vi "FPGA Host.vi"() -> (8 "FilePath":path=path "D:/temp/test.tdms")   [LabVIEW 2023]
uses:
  TypeDefs/WayPointCluster.ctl
  TypeDefs/Settings.ctl
  TypeDefs/ChangeOnFly.ctl
  TypeDefs/Display.ctl
  <vilib>/userDefined/High Color/nirio_resource_hc.ctl
  User_Vi/Settings.vi
  <vilib>/FPGAPlugInAG/PCIe-7856/niLvFpga_Open_PCIe-7856.vi
  <vilib>/FPGAPlugInAG/PCIe-7856/niLvFpga_Run_PCIe-7856.vi
  <vilib>/Utility/error.llb/Error Cluster From Error Code.vi
  <vilib>/rvi/errors/niLvFpgaAdjustHostInterfaceError.vi
  I32NonDim_to_umNonDim.vi
  <vilib>/rvi/interface/nirviOpenFPGA/nirviOpenFPGA.xnode
  TypeDefs/FPGA VI reference.ctl
  FPGA Bitfiles/wecspmpcie7856mi_FPGATarget2_FPGATargetPCIe78_PFpA9M1zUPQ.lvbitx
  <vilib>/rvi/interface/nirviMethod/nirviMethod.xnode
  <vilib>/rvi/interface/nirviReadWriteControl/nirviReadWriteControl.xnode
  <vilib>/rvi/errors/niLvFpgaMergeErrorWithErrorCode.vi
  NiFpgaLv.dll
  <vilib>/FPGAPlugInAG/PCIe-7856/niLvFpga_WriteFifo_PCIe-7856.vi
  <vilib>/FPGAPlugInAG/PCIe-7856/niLvFpga_ReadFifo_PCIe-7856.vi
  <vilib>/FPGAPlugInAG/PCIe-7856/niLvFpga_StartFifo_PCIe-7856.vi
  <vilib>/FPGAPlugInAG/PCIe-7856/niLvFpga_StopFifo_PCIe-7856.vi
panel:
  out "output cluster":T1
  out "DistanceToBulk":i16
  out "StopMoveV2":bool
  out "StopMoveV":bool
  out "StopMoveZ":bool
  out "StopMoveY":bool
  out "StopMoveX":bool
  out "Stop Hold Position":bool
  out "HoldTimer (ticks)":u64
  out "Feedback1 on  Hold":bool
  out "MeasuredCurrent":i16
  out "LineNumber":u64
  out "Feedback_Threshold":i32
  out "Feedback1 Error":i32
  out "Feedback1 Boolean":bool
  in  "Display Cluster":T2
  in  "ChangeonFly":T3
  in  "SettingsCluster":T4={"Sample Rate (us)"=1, "Samples Per Data Point (int, power of 2)"=1000, "DistanceToBulk (um)"=-1.0, "HoldTimeScaler"=1, "SaveData"=TRUE, "DistanceToBulk (um) 2"=-1.0, "DistanceToBulk (um) 3"=-1.0}
  in  "WayPointCluster":T5
  out "tdms file out":refnum<k34>
  out "ElementsToRead":u32=800
  in  "stop":bool
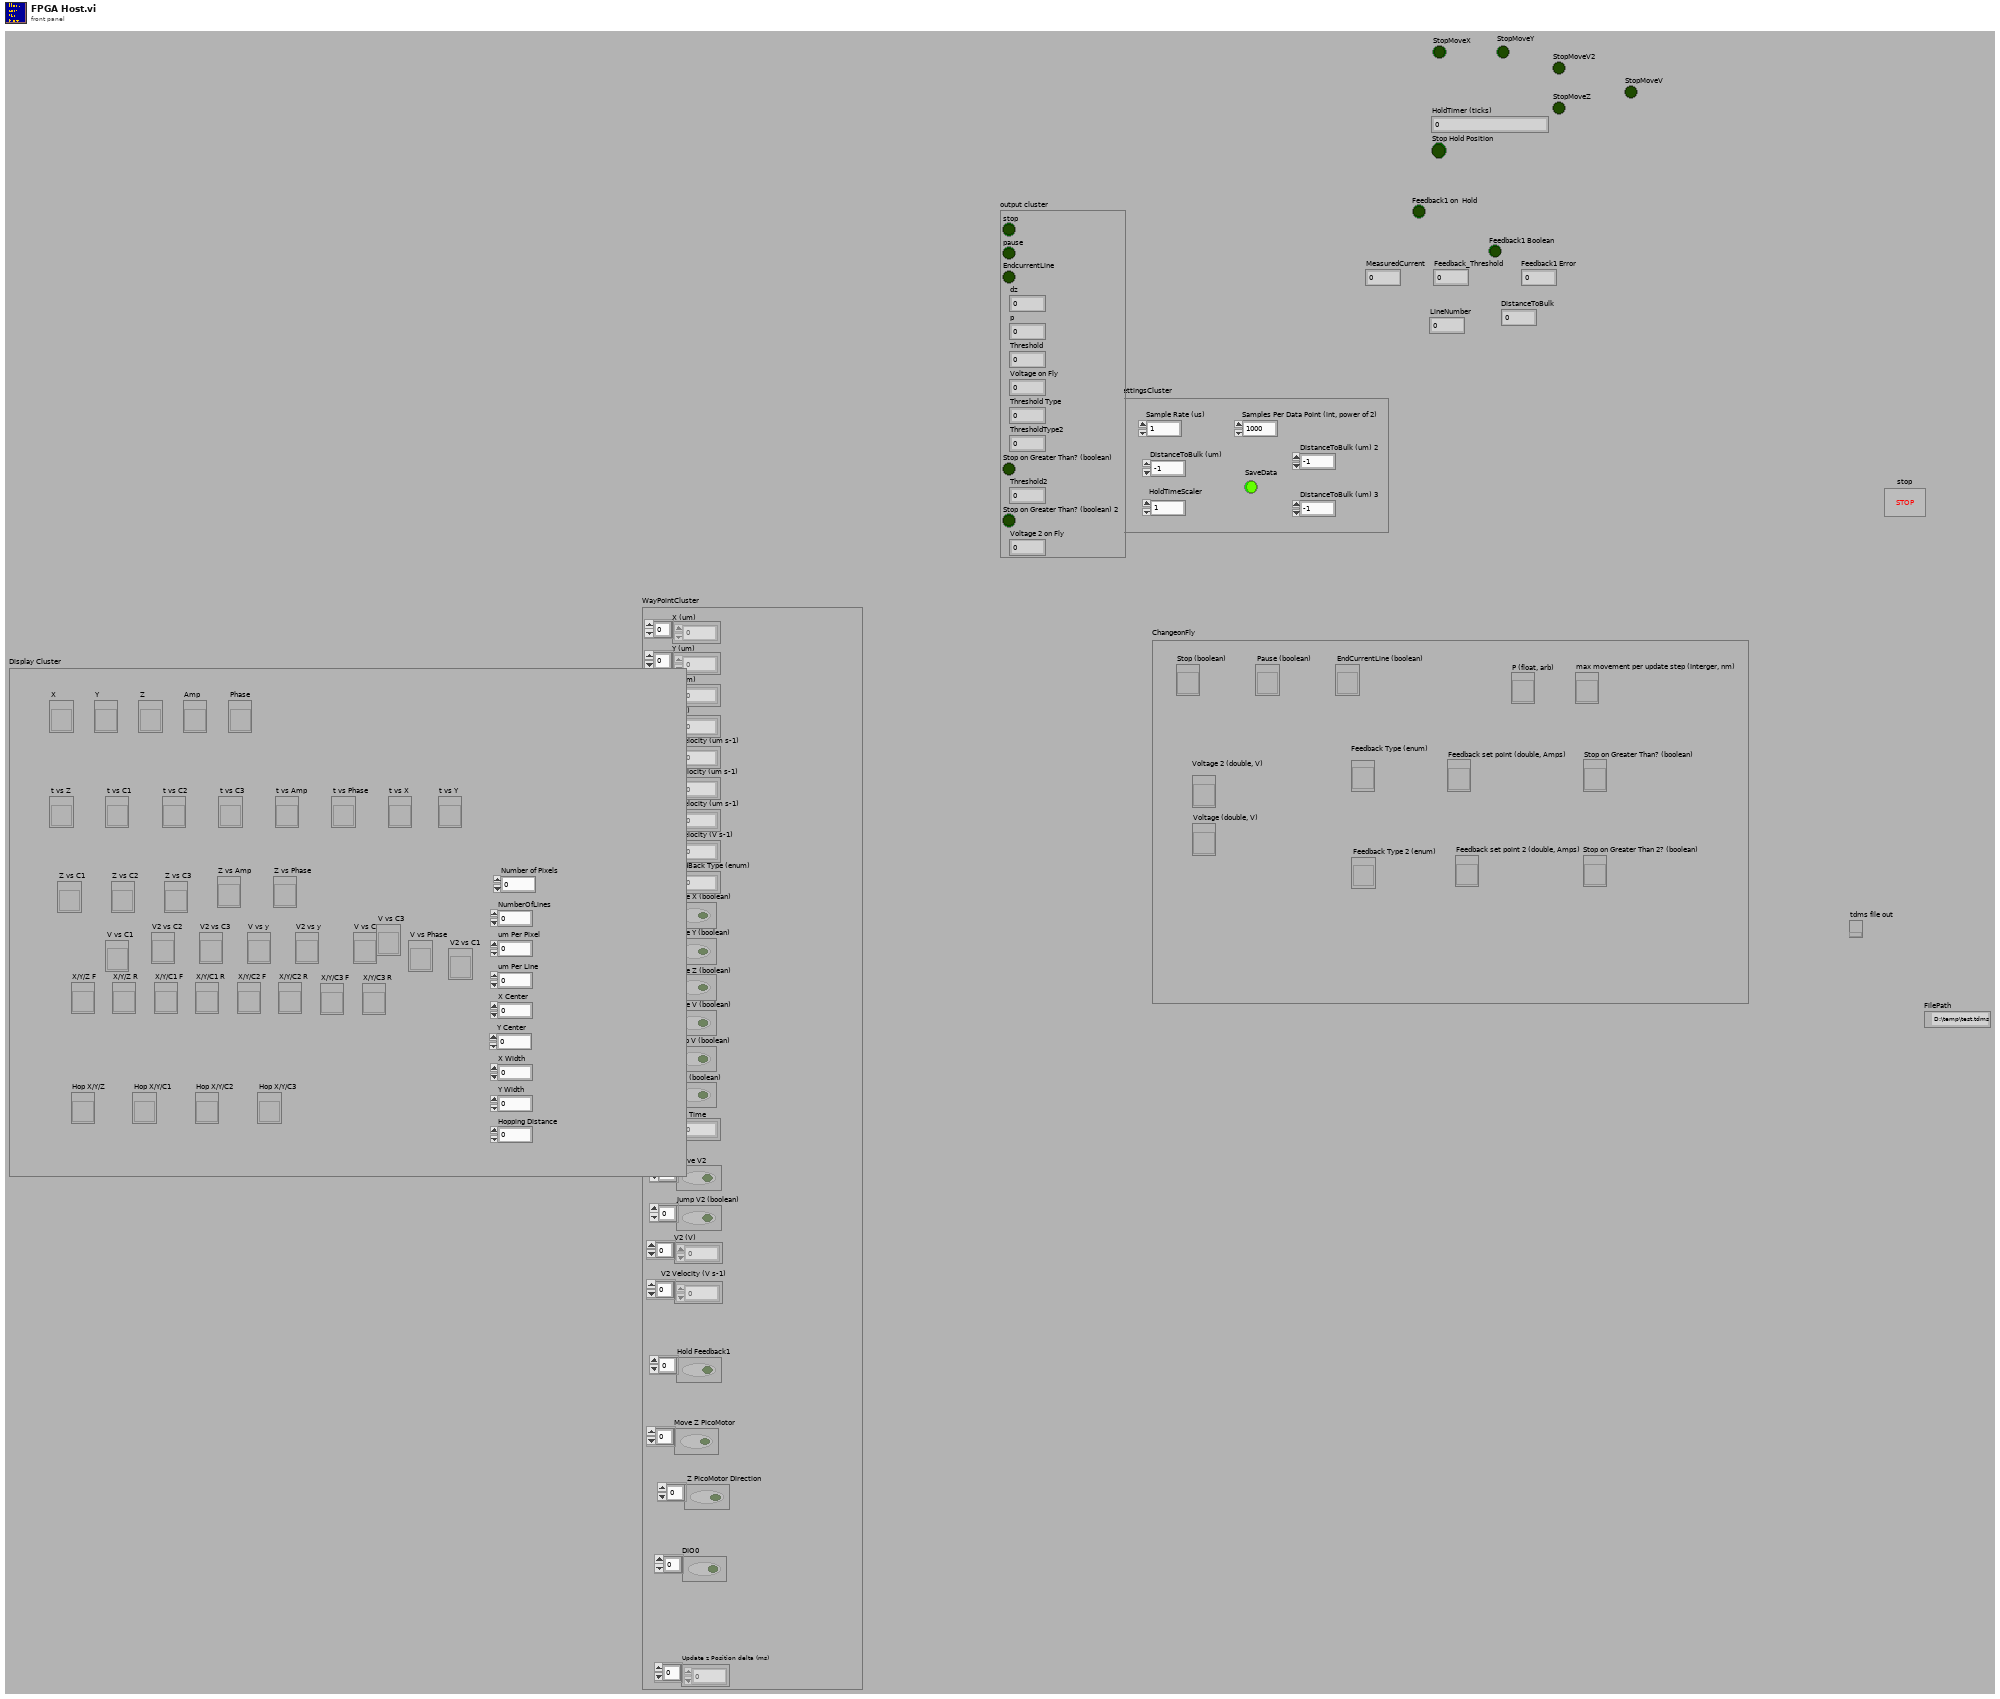
[diagram p1: front panel]
types:
  T1 = cluster{"stop":bool, "pause":bool, "EndcurrentLine":bool, "dz":i32, "p":fxp<+/-,32,1>, "Threshold":i64, "Voltage on Fly":i16, "Threshold Type":u8, "ThresholdType2":u8, "Stop on Greater Than? (boolean)":bool, "Threshold2":i64, "Stop on Greater Than? (boolean) 2":bool, "Voltage 2 on Fly":i16}
  T2 = typedef "Display.ctl" = cluster{"X":refnum<vi>, "Y":refnum<vi>, "Z":refnum<vi>, "Amp":refnum<vi>, "Phase":refnum<vi>, "t vs Z":refnum<vi>, "t vs C1":refnum<vi>, "t vs C2":refnum<vi>, "t vs C3":refnum<vi>, "t vs Amp":refnum<vi>, "t vs Phase":refnum<vi>, "t vs X":refnum<vi>, "t vs Y":refnum<vi>, "Z vs C1":refnum<vi>, "Z vs C2":refnum<vi>, "Z vs C3":refnum<vi>, "V vs C1":refnum<vi>, "V vs C2":refnum<vi>, "V vs C3":refnum<vi>, "X/Y/Z F":refnum<vi>, "X/Y/Z R":refnum<vi>, "X/Y/C1 F":refnum<vi>, "X/Y/C1 R":refnum<vi>, "X/Y/C2 F":refnum<vi>, "X/Y/C2 R":refnum<vi>, "X/Y/C3 F":refnum<vi>, "X/Y/C3 R":refnum<vi>, "NumberOfLines":u16, "um Per Pixel":dbl, "um Per Line":dbl, "X Center":dbl, "Hop X/Y/Z":refnum<vi>, "Hop X/Y/C1":refnum<vi>, "Hop X/Y/C2":refnum<vi>, "Hop X/Y/C3":refnum<vi>, "X Width":dbl, "Y Width":dbl, "Hopping Distance":dbl, "V2 vs C1":refnum<vi>, "V vs Phase":refnum<vi>, "Y Center":dbl, "Number of Pixels":dbl, "V2 vs C2":refnum<vi>, "V2 vs C3":refnum<vi>, "V vs y":refnum<vi>, "V2 vs y":refnum<vi>, "Z vs Amp":refnum<vi>, "Z vs Phase":refnum<vi>}
  T3 = typedef "ChangeOnFly.ctl" = cluster{"Stop (boolean)":refnum<vi>, "Pause (boolean)":refnum<vi>, "EndCurrentLine (boolean)":refnum<vi>, "max movement per update step (Interger, nm)":refnum<vi>, "P (float, arb)":refnum<vi>, "Feedback set point (double, Amps)":refnum<vi>, "Voltage (double, V)":refnum<vi>, "Feedback set point 2 (double, Amps)":refnum<vi>, "Stop on Greater Than 2? (boolean)":refnum<vi>, "Stop on Greater Than? (boolean)":refnum<vi>, "Voltage 2 (double, V)":refnum<vi>, "Feedback Type (enum)":refnum<vi>, "Feedback Type 2 (enum)":refnum<vi>}
  T4 = typedef "Settings.ctl" = cluster{"Sample Rate (us)":u32, "Samples Per Data Point (int, power of 2)":i16, "DistanceToBulk (um)":dbl, "HoldTimeScaler":u64, "SaveData":bool, "DistanceToBulk (um) 2":dbl, "DistanceToBulk (um) 3":dbl}
  T5 = typedef "WayPointCluster.ctl" = cluster{"X (um)":dbl[], "Y (um)":dbl[], "Z (um)":dbl[], "V (V)":dbl[], "X Velocity (um s-1)":dbl[], "Y Velocity (um s-1)":dbl[], "Z Velocity (um s-1)":dbl[], "V Velocity (V s-1)":dbl[], "FeedBack Type (enum)":u16[], "Move X (boolean)":bool[], "Move Y (boolean)":bool[], "Move Z (boolean)":bool[], "Move V (boolean)":bool[], "Jump V (boolean)":bool[], "Hold (boolean)":bool[], "Hold Time":u32[], "V2 (V)":dbl[], "Move V2":bool[], "V2 Velocity (V s-1)":dbl[], "Jump V2 (boolean)":bool[], "Update z Position delta (ms)":i16[], "Hold Feedback1":bool[], "Move Z PicoMotor":bool[], " Z PicoMotor Direction":bool[], "DIO0":bool[]}
  T6 = typedef "nirio_resource_hc.ctl" = tag
  T7 = typedef "FPGA VI reference.ctl" = refnum<k20>
  T8 = typedef "VelScallerCluster.ctl" = cluster{"X_VelScaller":i32, "Y_VelScaller":i32, "Z_VelScaller":i32, "V s-1_VelScaller":i32, "V2 s-1_VelScaller":i32}
  T9 = enum16{"open", "open or create", "create or replace", "create", "open (read-only)"}
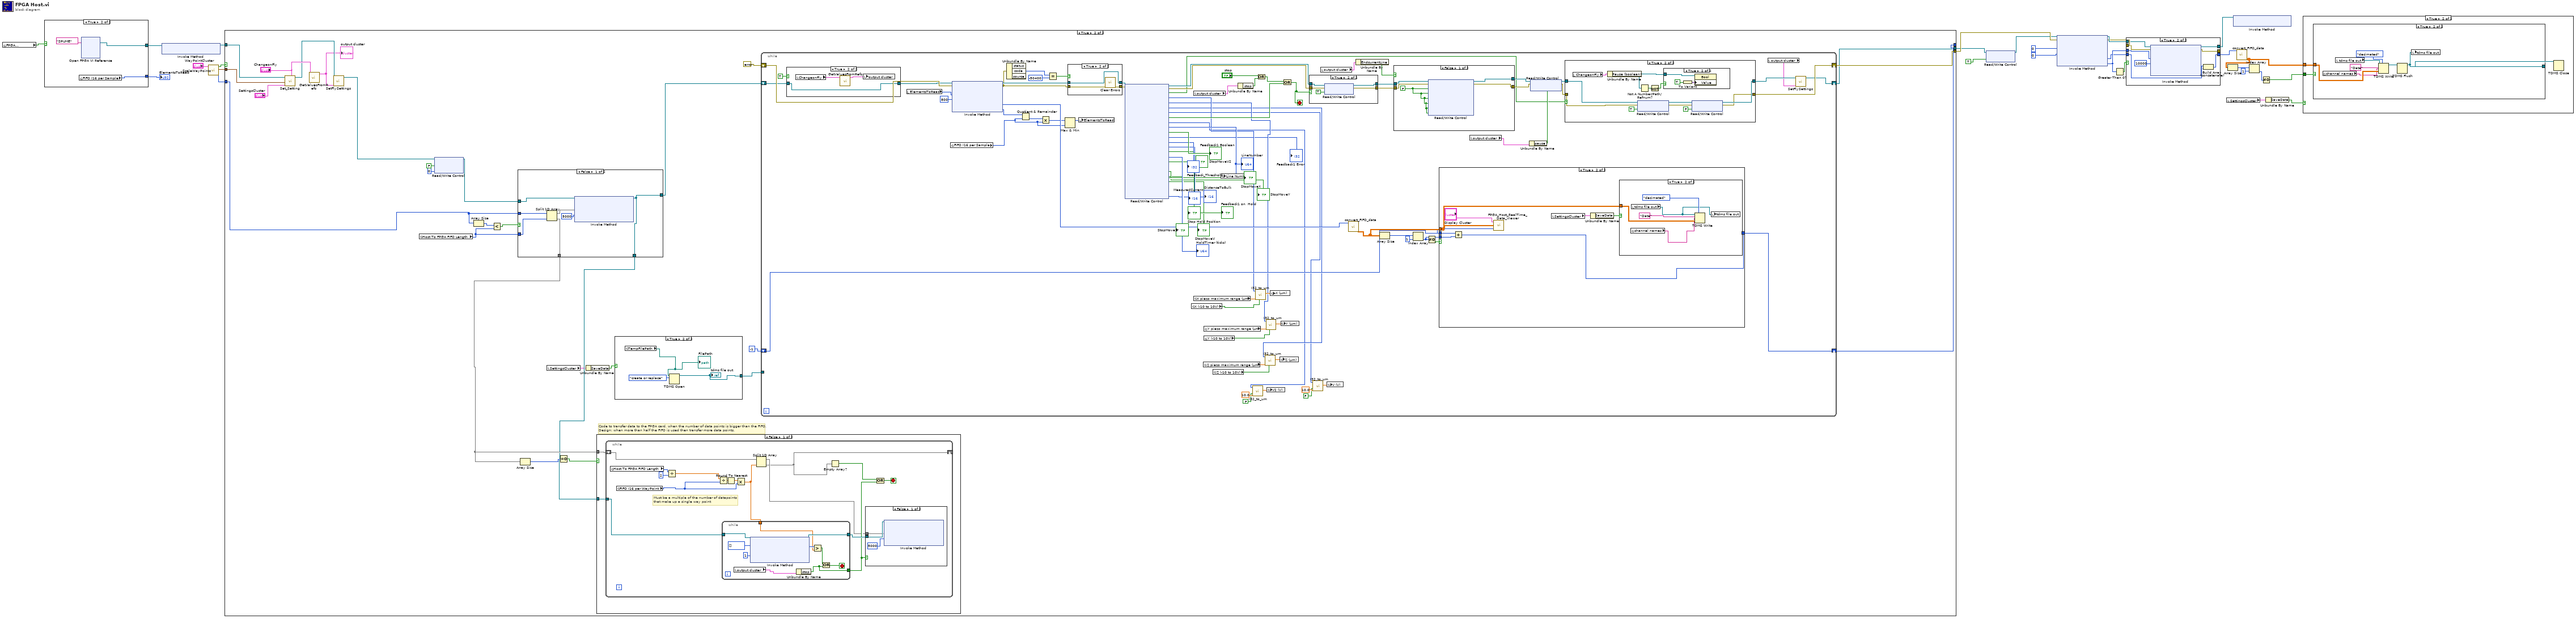
[diagram p0: block diagram]
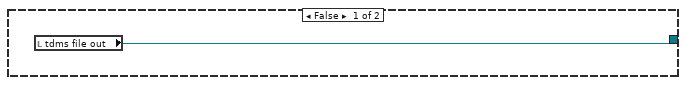
[diagram p3: hidden frame]
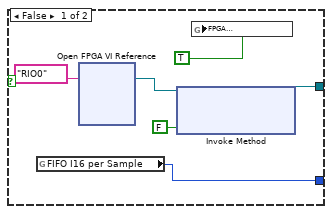
[diagram p4: hidden frame]
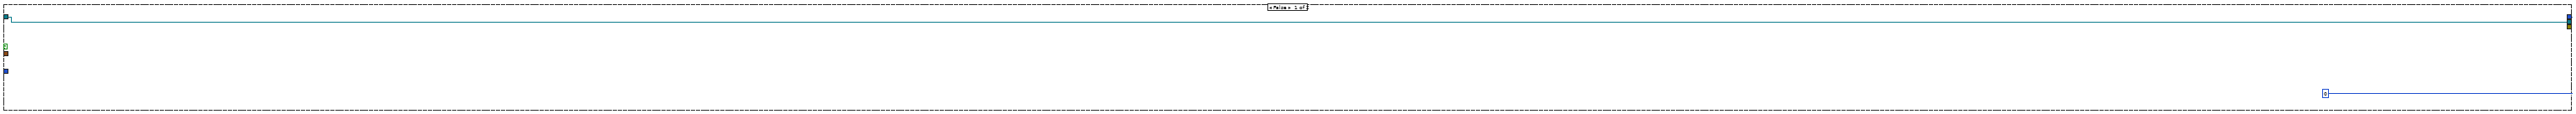
[diagram p6: hidden frame]
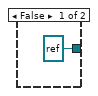
[diagram p7: hidden frame]
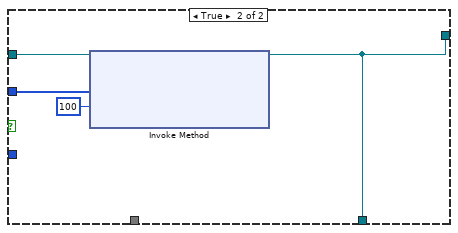
[diagram p10: hidden frame]
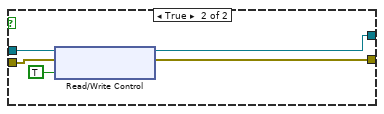
[diagram p14: hidden frame]
diagram:
  n1 = global read "Settings.vi" "FPGA \nrunning"() -> (w2:bool)
  n2 = case shown="True" w2 {
    tunnel: [w31 w36] -> w11
    tunnel: [w29 w35] -> w1
    frame False {
      n3 = global read "Settings.vi" "FIFO I16 per Sample"() -> (w29:u32)
      n4 = xnode "Open FPGA VI Reference"("resource name"=T6 "RIO0") -> ("FPGA VI Reference Out"=w32:T7)  [unwired: 1 in, 1 out]
      n5 = xnode "Invoke Method"("FPGA VI Reference In"=w32, "Wait Until Done (F)"=FALSE) -> ("FPGA VI Reference Out"=w31:T7)  [unwired: 1 in, 1 out]
      n6 = global write "Settings.vi" "FPGA \nrunning"(TRUE ("FPGA RUNNING")) -> ()
    }
    frame True {
      n7 = global read "Settings.vi" "FIFO I16 per Sample"() -> (w35:u32)
      n8 = xnode "Open FPGA VI Reference"("resource name"=T6 "SPUME") -> ("FPGA VI Reference Out"=w36:T7)  [unwired: 1 in, 1 out]
    }
  }
  "ElementsToRead" <- w1
  n9 = xnode "Invoke Method"("FPGA VI Reference In"=w11) -> ("FPGA VI Reference Out"=w10:T7)  [unwired: 1 in, 1 out]
  n10 = call "ScaleWayPoints.vi"("WayPointCluster"="WayPointCluster") -> ("FPGA Way Points"=w21:i16[], "VelScallerCluster"=w5:T8, ".not. x?"=w22:bool)  [unwired: 8 in]
  n11 = case shown="True" w22 {
    tunnel: [w38 w46] -> w8
    tunnel: [_ w66] -> w28
    tunnel: w21 -> [_ w55]
    tunnel: [0 ("dimension size") w60] -> _
    tunnel: w10 -> [w38 w48]
    tunnel: w5 -> [_ w44]
    frame False {
    }
    frame True {
      # "Code to transfer data to the FPGA card, when the number of data points is bigger than the FIFO.\nDesign: when more than half the FIFO is used then transfer more data points."
      n12 = call "Set_Setting.vi"("ChangeonFly"="ChangeonFly", "SettingsCluster"="SettingsCluster", "VelScallerCluster"=w44, "FPGA VI Reference Out 2"=w48) -> ("FPGA VI Reference Out 4"=w47:T7)  [unwired: 6 in, 1 out]
      n13 = call "GetValuesFromRefs.vi"("ChangeonFly"="ChangeonFly") -> ("output cluster"=w40:T1)  [unwired: 10 in]
      "output cluster" <- w40
      n14 = call "SetFlySettings.vi"("output cluster 4"=w40, "FPGA VI Reference Out 2"=w47) -> ("FPGA VI Reference Out 3"=w59:T7)  [unwired: 9 in]
      n15 = global read "Settings.vi" "Host To FPGA FIFO Length"() -> (w41:i64)
      n16 = xnode "Read/Write Control"("FPGA VI Reference In"=w59, "External Stop"=FALSE, "LineNumber"=0) -> ("FPGA VI Reference Out"=w58:T7)  [unwired: 1 in, 1 out]
      n17 = Array Size(array=w55) -> (size(s)=w54:i32)
      n18 = Less?(x=w54, y=w41) -> (x < y?=w53:bool)
      n19 = case shown="False" w53 {
        tunnel: w58 -> [w106 w111]
        tunnel: [w101 w108] -> w57
        tunnel: w55 -> [w105 w109]
        tunnel: w41 -> [w104 _]
        tunnel: [w102 _] -> w50
        tunnel: [w101 w108] -> w49
        frame False {
          n20 = Split 1D Array(array=w105, index=w104) -> (first subarray=w103:i16[], second subarray=w102:i16[])
          n21 = xnode "Invoke Method"("FPGA VI Reference In"=w106, "Data"=w103, "Timeout (ms)"=5000) -> ("FPGA VI Reference Out"=w101:T7)  [unwired: 1 in, 2 out]
        }
        frame True {
          n22 = xnode "Invoke Method"("FPGA VI Reference In"=w111, "Data"=w109, "Timeout (ms)"=100) -> ("FPGA VI Reference Out"=w108:T7)  [unwired: 1 in, 2 out]
        }
      }
      n23 = Array Size(array=w50) -> (size(s)=w52:i32)
      n24 = local read "SettingsCluster"() -> (w43:T4)
      n25 = Equal To 0?(x=w52) -> (x = 0?=w51:bool)
      n26 = Unbundle By Name(w43) -> ("SaveData"=w42:bool)
      n27 = case shown="False" w51 {
        tunnel: w50 -> [w72 _]
        tunnel: w49 -> [w71 _]
        frame False {
          n28 = while {
            shift-right: [w76] -> _
            shift-left: w72 -> [w87]
            tunnel: w71 -> [w79]
            stop <- w85 stop-if-true
            # "Must be a multiple of the number of datapoints \nthat make up a single way point"
            n29 = global read "Settings.vi" "Host To FPGA FIFO Length"() -> (w74:i64)
            n30 = global read "Settings.vi" "FIFO I16 per WayPoint"() -> (w73:i64)
            n31 = Divide(x=w74, y=i64 2) -> (x/y=w78:dbl)
            n32 = Divide(x=w78, y=w73) -> (x/y=w81:dbl)
            n33 = Round To Nearest(number=w81) -> (nearest integer value=w80:dbl)
            n34 = Multiply(x=w80, y=w73) -> (x*y=w77:dbl)
            n35 = while {
              tunnel: w79 -> [w95]
              tunnel: [w94] -> w84
              tunnel: [w98] -> w83
              tunnel: w77 -> [w92]
              stop <- w100 stop-if-true
              n36 = local read "output cluster"() -> (w91:T1)
              n37 = xnode "Invoke Method"("FPGA VI Reference In"=w95, "Data"=u64[] [], "Timeout (ms)"=1) -> ("FPGA VI Reference Out"=w94:T7, "Empty Elements Remaining"=w93:u32)  [unwired: 1 in, 1 out]
              n38 = Unbundle By Name(w91) -> ("stop"=w98:bool)
              n39 = Greater?(x=w93, y=w92) -> (0:w99:bool)
              n40 = Or(x=w99, y=w98) -> (x .or. y?=w100:bool)
            }
            n41 = Split 1D Array(array=w87, index=w77) -> (first subarray=w82:i16[], second subarray=w76:i16[])
            n42 = Empty Array?(array=w76) -> (empty?=w75:bool)
            n43 = case shown="False" w83 {
              tunnel: w84 -> [w89 _]
              tunnel: w82 -> [w88 _]
              frame False {
                n44 = xnode "Invoke Method"("FPGA VI Reference In"=w89, "Data"=w88, "Timeout (ms)"=5000) -> ()  [unwired: 1 in, 3 out]
              }
              frame True {
              }
            }
            n45 = Or(x=w75, y=w83) -> (x .or. y?=w85:bool)
          }
        }
        frame True {
        }
      }
      n46 = case shown="True" w42 {
        tunnel: [refnum<k34> refnum ("tdms file out") w70] -> w64
        frame False {
        }
        frame True {
          n47 = global read "Settings.vi" "TempFilePath"() -> (w68:path)
          "FilePath" <- w68
          n48 = TDMS Open(10:T9."create or replace" ("operation (0:open)"), 11:w68) -> (3:w70:refnum<k34>)  [unwired: 5 in, 1 out]
          "tdms file out" <- w70
        }
      }
      n49 = while {
        shift-right: [w155] -> w66
        shift-left: errorcluster {"status"=FALSE, "code"=0, "source"=""} ("error out") -> [w193]
        shift-right: [w133] -> w46
        shift-left: w57 -> [w160]
        shift-right: [w178] -> w60
        shift-left: -1 ("dimension size") -> [w188]
        tunnel: w64 -> [_]
        stop <- w154 stop-if-true
        n50 = case shown="True" TRUE {
          tunnel: w160 -> [w195 w198]
          tunnel: [w195 w198] -> w159
          frame False {
          }
          frame True {
            n51 = local read "ChangeonFly"() -> (w197:T3)
            n52 = call "GetValuesFromRefs.vi"("ChangeonFly"=w197) -> ("output cluster"=w196:T1)  [unwired: 10 in]
            n53 = local write "output cluster"(w196) -> ()
          }
        }
        n54 = local read "ElementsToRead"() -> (w180:u32)
        n55 = global read "Settings.vi" "FIFO I16 per Sample"() -> (w120:u32)
        n56 = xnode "Invoke Method"("FPGA VI Reference In"=w159, "error in"=w193, "Number of Elements"=w180, "Timeout (ms)"=800) -> ("FPGA VI Reference Out"=w182:T7, "error out"=w181:errorcluster, "Data"=w189:i16[], "Elements Remaining"=w179:u32)
        n57 = Unbundle By Name(w181) -> ("code"=w192:i32)  [unwired: 2 out]
        n58 = Quotient & Remainder(x=w179, y=w120) -> (floor(x/y)=w175:u32)  [unwired: 1 out]
        n59 = Multiply(x=w175, y=w120) -> (x*y=w177:u32)
        n60 = Equal?(x=w192, y=-50400) -> (x = y?=w190:bool)
        n61 = Max & Min(x=w177, y=w120) -> (max(x,y)=w176:u32)  [unwired: 1 out]
        n62 = case shown="True" w190 {
          tunnel: w181 -> [w247 w250]
          tunnel: [w247 w249] -> w186
          tunnel: w182 -> [w246 w248]
          tunnel: [w246 w248] -> w185
          frame False {
          }
          frame True {
            n63 = call <vilib>:"Clear Errors.vi"("error in (no error)"=w250) -> ("error out"=w249:errorcluster)  [unwired: 5 in, 1 out]
          }
        }
        n64 = local write "ElementsToRead"(w176) -> ()
        n65 = xnode "Read/Write Control"("FPGA VI Reference In"=w185, "error in"=w186) -> ("FPGA VI Reference Out"=w184:T7, "error out"=w183:errorcluster, "Internal Pause"=w157:bool, "Applied X"=w150:i16, "Applied Y"=w148:i16, "Applied Z"=w143:i16, "Applied Voltage"=w141:i16, "WaitingForWayPoints"=w153:bool, "Applied Voltage 2"=w138:i16, "LineNumber"=w152:u64, "Feedback1 Boolean"=→"Feedback1 Boolean":bool, "Feedback1 Error"=→"Feedback1 Error":i32, "Feedback_Threshold"=→"Feedback_Threshold":i64, "MeasuredCurrent"=→"MeasuredCurrent":i16, "Feedback1 on  Hold"=→"Feedback1 on  Hold":bool, "HoldTimer (ticks)"=→"HoldTimer (ticks)":u64, "Stop Hold Position"=→"Stop Hold Position":bool, "StopMoveX"=→"StopMoveX":bool, "StopMoveY"=→"StopMoveY":bool, "StopMoveZ"=→"StopMoveZ":bool, "StopMoveV"=→"StopMoveV":bool, "StopMoveV2"=→"StopMoveV2":bool, "DistanceToBulk"=→"DistanceToBulk":i16)  [unwired: 1 out]
        "LineNumber" <- w152
        n66 = global read "Settings.vi" "X (-10 to 10V)"() -> (w119:bool)
        n67 = local read "output cluster"() -> (w112:T1)
        n68 = global read "Settings.vi" "X piezo maximum range (µm)"() -> (w149:dbl)
        n69 = global read "Settings.vi" "Z piezo maximum range (µm)"() -> (w144:dbl)
        n70 = global read "Settings.vi" "Y piezo maximum range (µm)"() -> (w147:dbl)
        n71 = global read "Settings.vi" "Y (-10 to 10V)"() -> (w118:bool)
        n72 = global read "Settings.vi" "Z (-10 to 10V)"() -> (w117:bool)
        n73 = global write "Settings.vi" "Line Number"(w152) -> ()
        n74 = Unbundle By Name(w112) -> ("stop"=w167:bool)
        n75 = call-poly "I32_to_um.vi"("-10 to 10V range?"=FALSE, "Max Value [um]"=10.0 ("n"), "Input"=w138) -> ("x*y"=w137:dbl)  [unwired: 8 in]
        n76 = call-poly "I32_to_um.vi"("-10 to 10V range?"=w119, "Max Value [um]"=w149, "Input"=w150) -> ("x*y"=w151:dbl)  [unwired: 8 in]
        n77 = Or(x="stop", y=w167) -> (x .or. y?=w166:bool)
        n78 = call-poly "I32_to_um.vi"("-10 to 10V range?"=w117, "Max Value [um]"=w144, "Input"=w143) -> ("x*y"=w145:dbl)  [unwired: 8 in]
        n79 = call-poly "I32_to_um.vi"("-10 to 10V range?"=w118, "Max Value [um]"=w147, "Input"=w148) -> ("x*y"=w146:dbl)  [unwired: 8 in]
        n80 = global write "Settings.vi" "V2 (V)"(w137) -> ()
        n81 = global write "Settings.vi" "X (µm)"(w151) -> ()
        n82 = global write "Settings.vi" "Z (µm)"(w145) -> ()
        n83 = global write "Settings.vi" "Y (µm)"(w146) -> ()
        n84 = Or(x=w166, y=w153) -> (x .or. y?=w154:bool)
        n85 = case shown="True" w154 {
          tunnel: [w239 w245] -> w170
          tunnel: [w240 w244] -> w168
          tunnel: w183 -> [w240 w243]
          tunnel: w184 -> [w239 w241]
          frame False {
          }
          frame True {
            n86 = xnode "Read/Write Control"("FPGA VI Reference In"=w241, "error in"=w243, "External Stop"=TRUE ("Stop")) -> ("FPGA VI Reference Out"=w245:T7, "error out"=w244:errorcluster)
          }
        }
        n87 = call-poly "I32_to_um.vi"("-10 to 10V range?"=FALSE, "Max Value [um]"=10.0 ("n"), "Input"=w141) -> ("x*y"=w140:dbl)  [unwired: 8 in]
        n88 = local read "output cluster"() -> (w115:T1)
        n89 = global write "Settings.vi" "V (V)"(w140) -> ()
        n90 = call "convert_FIFO_data.vi"("Actual Data"=w189) -> ("appended array"=w156:dbl[][])  [unwired: 18 in]
        n91 = Unbundle By Name(w115) -> ("EndcurrentLine"=w165:bool)
        n92 = Array Size(array=w156) -> (size(s)=w174:i32[])
        n93 = case shown="False" w165 {
          tunnel: w170 -> [w220 w225]
          tunnel: [w219 w224] -> w169
          tunnel: w168 -> [w218 w223]
          tunnel: [w217 w222] -> w162
          frame False {
            w216 = FALSE ("OnlyStopLineONCE")
            n94 = xnode "Read/Write Control"("FPGA VI Reference In"=w220, "error in"=w218, "OnlyStopLineONCE V"=w216, "OnlyStopLineONCE Z"=w216, "OnlyStopLineONCE Y"=w216, "OnlyStopLineONCE X"=w216, "EndCurrentLine"=w216, "OnlyStopLineONCE V2"=w216) -> ("FPGA VI Reference Out"=w219:T7, "error out"=w217:errorcluster)
          }
          frame True {
            n95 = xnode "Read/Write Control"("FPGA VI Reference In"=w225, "error in"=w223, "EndCurrentLine"=TRUE) -> ("FPGA VI Reference Out"=w224:T7, "error out"=w222:errorcluster)
          }
        }
        n96 = Index Array(array=w174, index=1) -> (element=w171:i32)
        n97 = Not Equal To 0?(x=w171) -> (x != 0?=w172:bool)
        n98 = case shown="True" w172 {
          tunnel: w188 -> [w226 w232]
          tunnel: [w226 w231] -> w178
          tunnel: w156 -> [_ w229]
          tunnel: w171 -> [_ w233]
          frame False {
          }
          frame True {
            n99 = Add(x=w232, y=w233) -> (x+y=w231:i32)
            n100 = call "FPGA_Host_RealTime_Data_Viewer.vi"("length"=w232, "Array"=w229, "Display Cluster"="Display Cluster") -> ()  [unwired: 3 in]
            n101 = local read "SettingsCluster"() -> (w228:T4)
            n102 = Unbundle By Name(w228) -> ("SaveData"=w227:bool)
            n103 = case shown="True" w227 {
              tunnel: w229 -> [_ w238]
              frame False {
              }
              frame True {
                n104 = global read "Settings.vi" "channel names"() -> (w235:string[])
                n105 = local read "tdms file out"() -> (w234:refnum<k34>)
                n106 = TDMS Write(0:w234, 1:enum16{"decimated", "interleaved"}."decimated" ("data layout (0:decimated)"), 5:"Data" ("group name in (Untitled)"), 7:w235, 9:w238) -> ()  [unwired: 1 in, 4 out]
                n107 = local write "tdms file out"(w234) -> ()
              }
            }
          }
        }
        n108 = local read "output cluster"() -> (w114:T1)
        n109 = Unbundle By Name(w114) -> ("pause"=w163:bool)
        n110 = xnode "Read/Write Control"("FPGA VI Reference In"=w169, "error in"=w162, "External Pause"=w163) -> ("FPGA VI Reference Out"=w164:T7, "error out"=w161:errorcluster)
        n111 = case shown="True" w157 {
          tunnel: w164 -> [w200 w212]
          tunnel: [w200 w209] -> w134
          tunnel: w161 -> [w199 w207]
          tunnel: [w199 w205] -> w155
          frame False {
          }
          frame True {
            n112 = local read "ChangeonFly"() -> (w201:T3)
            n113 = Unbundle By Name(w201) -> ("Pause (boolean)"=w203:refnum<vi>)
            n114 = xnode "Read/Write Control"("FPGA VI Reference In"=w212, "error in"=w207, "External Pause"=TRUE) -> ("FPGA VI Reference Out"=w210:T7, "error out"=w206:errorcluster)
            n115 = Not A Number/Path/Refnum?(number/path/refnum=w203) -> (NaN/Path/Refnum?=w204:bool)
            n116 = Not(x=w204) -> (.not. x?=w202:bool)
            n117 = case shown="True" w202 {
              tunnel: w203 -> [_ w213]
              frame False {
              }
              frame True {
                n118 = To Variant(anything=TRUE) -> (Variant=w214:variant)
                n119 = property on="Property Node" class="Bool"(reference=w213, "Value"=w214) -> ()  [unwired: 1 in, 2 out]
              }
            }
            n120 = xnode "Read/Write Control"("FPGA VI Reference In"=w210, "error in"=w206, "Internal Pause"=FALSE) -> ("FPGA VI Reference Out"=w209:T7, "error out"=w205:errorcluster)
          }
        }
        n121 = local read "output cluster"() -> (w113:T1)
        n122 = call "SetFlySettings.vi"("output cluster 4"=w113, "FPGA VI Reference Out 2"=w134) -> ("FPGA VI Reference Out 3"=w133:T7)  [unwired: 9 in]
      }
    }
  }
  n123 = xnode "Read/Write Control"("FPGA VI Reference In"=w8, "External Stop"=TRUE) -> ("FPGA VI Reference Out"=w6:T7)  [unwired: 1 in, 1 out]
  n124 = xnode "Invoke Method"("FPGA VI Reference In"=w6, "error in"=w28, "Number of Elements"=u32 0, "Timeout (ms)"=0) -> ("FPGA VI Reference Out"=w19:T7, "error out"=w14:errorcluster, "Data"=w23:i16[], "Elements Remaining"=w24:u32)
  n125 = Greater Than 0?(x=w24) -> (x > 0?=w25:bool)
  n126 = case shown="True" w25 {
    tunnel: w19 -> [w251 w262]
    tunnel: w24 -> [_ w261]
    tunnel: w23 -> [w253 w259]
    tunnel: [w253 w257] -> w20
    tunnel: w14 -> [w252 w256]
    tunnel: [w252 w255] -> _
    tunnel: [w251 w254] -> w12
    frame False {
    }
    frame True {
      n127 = xnode "Invoke Method"("FPGA VI Reference In"=w262, "error in"=w256, "Number of Elements"=w261, "Timeout (ms)"=10000) -> ("FPGA VI Reference Out"=w254:T7, "error out"=w255:errorcluster, "Data"=w258:i16[])  [unwired: 1 out]
      n128 = Build Array (concatenate)(w259, w258) -> (w257:i16[])
    }
  }
  n129 = local read "SettingsCluster"() -> (w4:T4)
  n130 = xnode "Invoke Method"("FPGA VI Reference In"=w12) -> ()  [unwired: 1 in, 2 out]
  n131 = call "convert_FIFO_data.vi"("Actual Data"=w20) -> ("appended array"=w13:dbl[][])  [unwired: 18 in]
  n132 = Array Size(array=w13) -> (size(s)=w18:i32[])
  n133 = Index Array(array=w18, index=1) -> (element=w16:i32)
  n134 = Not Equal To 0?(x=w16) -> (x != 0?=w15:bool)
  n135 = Unbundle By Name(w4) -> ("SaveData"=w3:bool)
  n136 = case shown="True" w3 {
    tunnel: w15 -> [_ w265]
    tunnel: w13 -> [_ w264]
    frame False {
    }
    frame True {
      n137 = case shown="True" w265 {
        tunnel: w264 -> [_ w273]
        tunnel: [w266 w268] -> w263
        frame False {
          n138 = local read "tdms file out"() -> (w266:refnum<k34>)
        }
        frame True {
          n139 = global read "Settings.vi" "channel names"() -> (w267:string[])
          n140 = local read "tdms file out"() -> (w271:refnum<k34>)
          n141 = TDMS Write(0:w271, 1:enum16{"decimated", "interleaved"}."decimated" ("data layout (0:decimated)"), 5:"Data" ("group name in (Untitled)"), 7:w267, 9:w273) -> (4:w270:refnum<k34>)  [unwired: 1 in, 3 out]
          n142 = TDMS Flush(7:w270) -> (3:w268:refnum<k34>)  [unwired: 1 in, 1 out]
          n143 = local write "tdms file out"(w268) -> ()
        }
      }
      n144 = TDMS Close(11:w263) -> ()  [unwired: 1 in, 2 out]
    }
  }
